vi "sub_LV_GraphController.vi"(8 "Number of samples":i32, 10 "Input sample":dbl, 11 "Prev. data":dbl[](array[numeric])) -> (3 "Graph data":dbl[](array[numeric]))   [LabVIEW 2012]
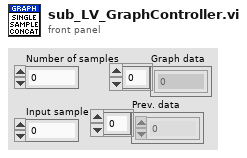
[diagram p1: front panel]
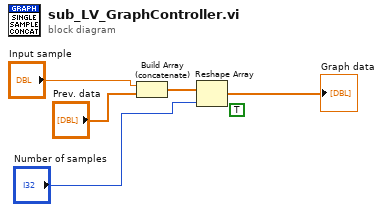
[diagram p0: block diagram]
diagram:
  (unwired) TRUE
  n1 = Build Array (concatenate)("Input sample", "Prev. data") -> (w2:dbl[])
  n2 = Reshape Array(w2, "Number of samples") -> (→"Graph data":dbl[])
